vi "LCR_ReadMType.vi"(8 "error in (no error)":errorcluster, 10 "Configuration Cluster":T1={"General"={"Config.ini"=path "", "Default Logging Path"=path ""}, "Hardware"={"AHC VISA COM"="", "Measure Rate (1/s)"=0, "Global T VAR"="", "Global B VAR"=""}, "Operation"={"Operation Mode"=enum."Idle-Off", "Status"="", "NewLog?"=FALSE}}) -> (0 "error out":errorcluster, 2 "Configuration Cluster Out":T1={"General"={"Config.ini"=path "", "Default Logging Path"=path ""}, "Hardware"={"AHC VISA COM"="", "Measure Rate (1/s)"=0, "Global T VAR"="", "Global B VAR"=""}, "Operation"={"Operation Mode"=enum."Idle-Off", "Status"="", "NewLog?"=FALSE}}, 4 "Secondary Unit":T3, 6 "Primary Unit":T3)   [LabVIEW 2021]
uses:
  UnitEnum.ctl
  Mode_Enum.ctl
  Config_Cluster.ctl
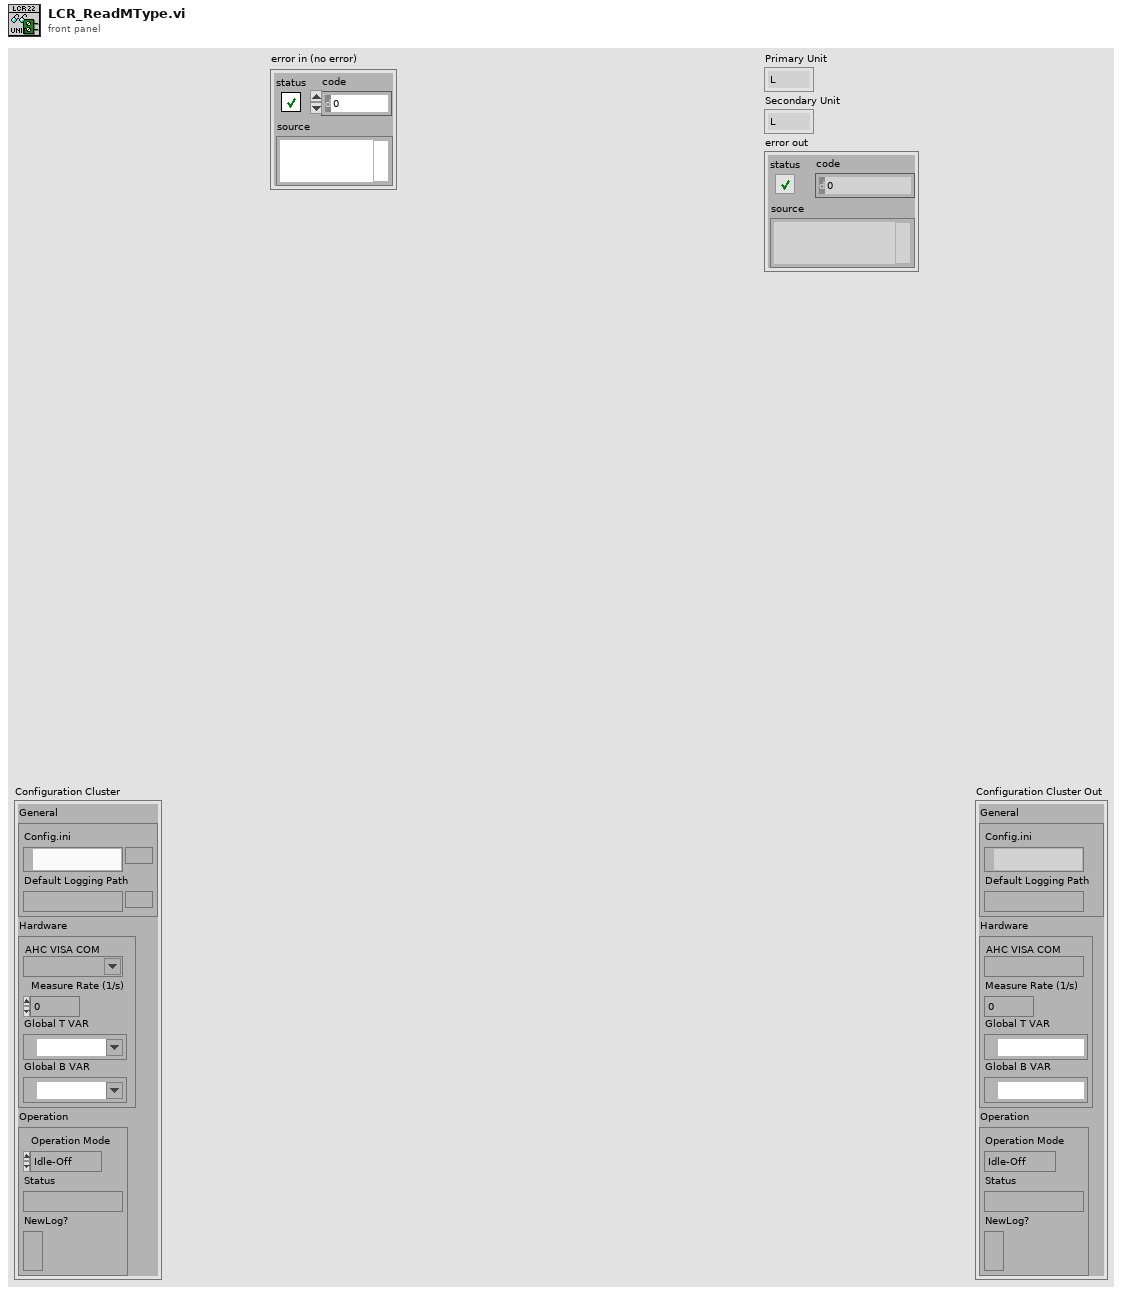
[diagram p1: front panel]
types:
  T1 = typedef "Config_Cluster.ctl" = cluster{"General":cluster{"Config.ini":path, "Default Logging Path":path}, "Hardware":cluster{"AHC VISA COM":refnum<visa-resource-name>, "Measure Rate (1/s)":i32, "Global T VAR":refnum<k21>, "Global B VAR":refnum<k21>}, "Operation":cluster{"Operation Mode":T2, "Status":string, "NewLog?":bool}}
  T2 = typedef "Mode_Enum.ctl" = enum16{"Logging", "Idle-Off", "Idle"}
  T3 = typedef "UnitEnum.ctl" = enum16{"L", "R", "C", "Z", "X", "Q", "Theta", "Y", "N", "M", "G", "B", "D"}
  T4 = enum16{"Auto", "L-Q", "L-R", "C-D", "C-R", "R-Q", "Z-Theta", "Y+Theta", "R+X", "G+B", "N+Theta", "M"}
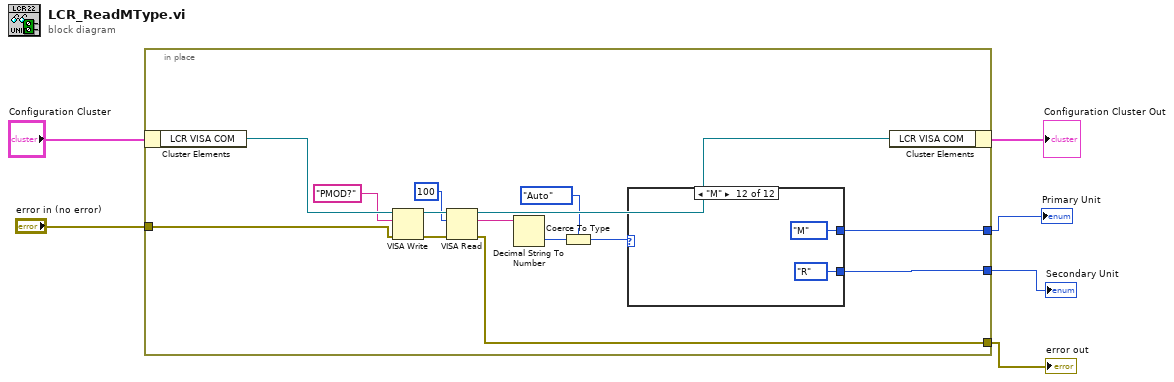
[diagram p0: block diagram]
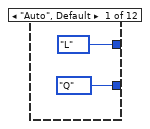
[diagram p2: hidden frame]
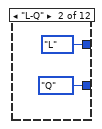
[diagram p3: hidden frame]
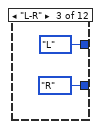
[diagram p4: hidden frame]
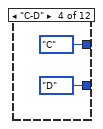
[diagram p5: hidden frame]
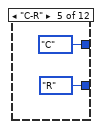
[diagram p6: hidden frame]
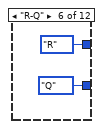
[diagram p7: hidden frame]
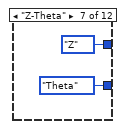
[diagram p8: hidden frame]
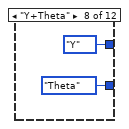
[diagram p9: hidden frame]
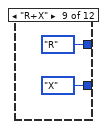
[diagram p10: hidden frame]
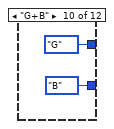
[diagram p11: hidden frame]
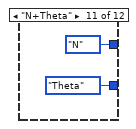
[diagram p12: hidden frame]
diagram:
  n1 = in-place {
    in-place-border: "error in (no error)" -> [w18]
    in-place-border: [w9] -> w4
    in-place-border: [w8] -> w3
    in-place-border: [w7] -> w2
    n2 = in-place-cluster #1("Configuration Cluster") -> ("LCR VISA COM"=w20:refnum<visa-resource-name>)
    n3 = VISA Write(VISA resource name=w20, write buffer="PMOD?", error in (no error)=w18) -> (VISA resource name out=w16:refnum<visa-resource-name>, error out=w17:errorcluster)  [unwired: 1 out]
    n4 = VISA Read(VISA resource name=w16, byte count=u32 100, error in (no error)=w17) -> (VISA resource name out=w14:refnum<visa-resource-name>, read buffer=w13:string, error out=w7:errorcluster)  [unwired: 1 out]
    n5 = Decimal String To Number(string=w13) -> (number=w12:i32)  [unwired: 2 in, 1 out]
    n6 = Coerce To Type(0:w12, 1:T4."Auto") -> (2:w10:T4)
    n7 = case shown="\"M\"" w10 {
      tunnel: [UnitEnum."L" UnitEnum."L" UnitEnum."L" UnitEnum."C" UnitEnum."C" UnitEnum."R" UnitEnum."Z" UnitEnum."Y" UnitEnum."R" UnitEnum."G" UnitEnum."N" UnitEnum."M"] -> w9
      tunnel: [UnitEnum."Q" UnitEnum."Q" UnitEnum."R" UnitEnum."D" UnitEnum."R" UnitEnum."Q" UnitEnum."Theta" UnitEnum."Theta" UnitEnum."X" UnitEnum."B" UnitEnum."Theta" UnitEnum."R"] -> w8
      frame "Auto", Default {
      }
      frame "L-Q" {
      }
      frame "L-R" {
      }
      frame "C-D" {
      }
      frame "C-R" {
      }
      frame "R-Q" {
      }
      frame "Z-Theta" {
      }
      frame "Y+Theta" {
      }
      frame "R+X" {
      }
      frame "G+B" {
      }
      frame "N+Theta" {
      }
      frame "M" {
      }
    }
    n8 = in-place-cluster #1("LCR VISA COM"=w14) -> (→"Configuration Cluster Out":T1)
  }
  "Primary Unit" <- w4
  "Secondary Unit" <- w3
  "error out" <- w2
